vi "PSCreatePngChunk.vi"(10 "Data":string, 11 "Name":string) -> (3 "PNG Chunk":string)   [LabVIEW 2013]
doc: "Ceates a PNG chunk.\nCode by Darin"
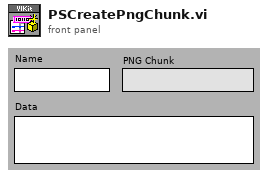
[diagram p1: front panel]
types:
  T1 = enum16{"Make CRC Table", "CRC", "Update_CRC_C", "Update_CRC_S"}
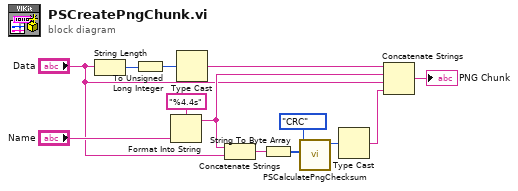
[diagram p0: block diagram]
diagram:
  n1 = String Length(string="Data") -> (length=w13:i32)
  n2 = To Unsigned Long Integer(number=w13) -> (unsigned 32bit integer=w12:u32)
  n3 = Format Into String(format string="%4.4s", "Name") -> (resulting string=w3:string)  [unwired: 2 in, 1 out]
  n4 = Type Cast(x=w12) -> (*(type *) &x=w9:string)  [unwired: 1 in]
  n5 = Concatenate Strings(w3, "Data") -> (w2:string)
  n6 = String To Byte Array(string=w2) -> (unsigned byte array=w8:u8[])
  n7 = call "PSCalculatePngChecksum.vi"("Byte Array"=w8, "Operation"=T1."CRC") -> ("CRC"=w6:u32)  [unwired: 8 in, 1 out]
  n8 = Type Cast(x=w6) -> (*(type *) &x=w5:string)  [unwired: 1 in]
  n9 = Concatenate Strings(w9, w3, "Data", w5) -> (→"PNG Chunk":string)
